vi "New Frame Trigger.vi"(8 "error in":errorcluster, 10 "Trigger":bool, 11 "CaptureDetectionLoopDataIn":T1={"Captures"=path "", "Timeout"=-1, "Reset"=TRUE, "Trigger"=FALSE, "Iteration"=0, "Capture"=path "", "Mode"=enum."Record", "Replay Run ID"=""}) -> (0 "error out":errorcluster, 2 "Latest Frame":path, 3 "CaptureDetectionLoopDataOut":T1={"Captures"=path "", "Timeout"=-1, "Reset"=TRUE, "Trigger"=FALSE, "Iteration"=0, "Capture"=path "", "Mode"=enum."Record", "Replay Run ID"=""})   [LabVIEW 2026, in "Launcher.lvlib"]
uses:
  Launcher.lvlib
  Capture detection loop data--cluster.ctl
  Mode.ctl
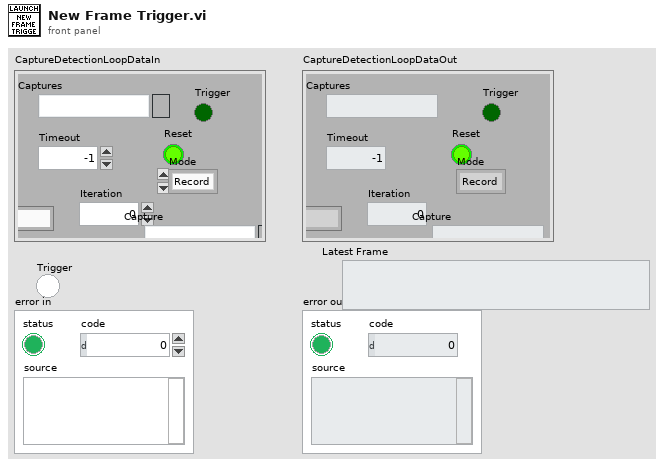
[diagram p1: front panel]
types:
  T1 = typedef "Capture detection loop data--cluster.ctl" = cluster{"Captures":path, "Timeout":i32, "Reset":bool, "Trigger":bool, "Iteration":i32, "Capture":path, "Mode":T2, "Replay Run ID":string}
  T2 = typedef "Mode.ctl" = enum16{"Record", "Record and Replay"}
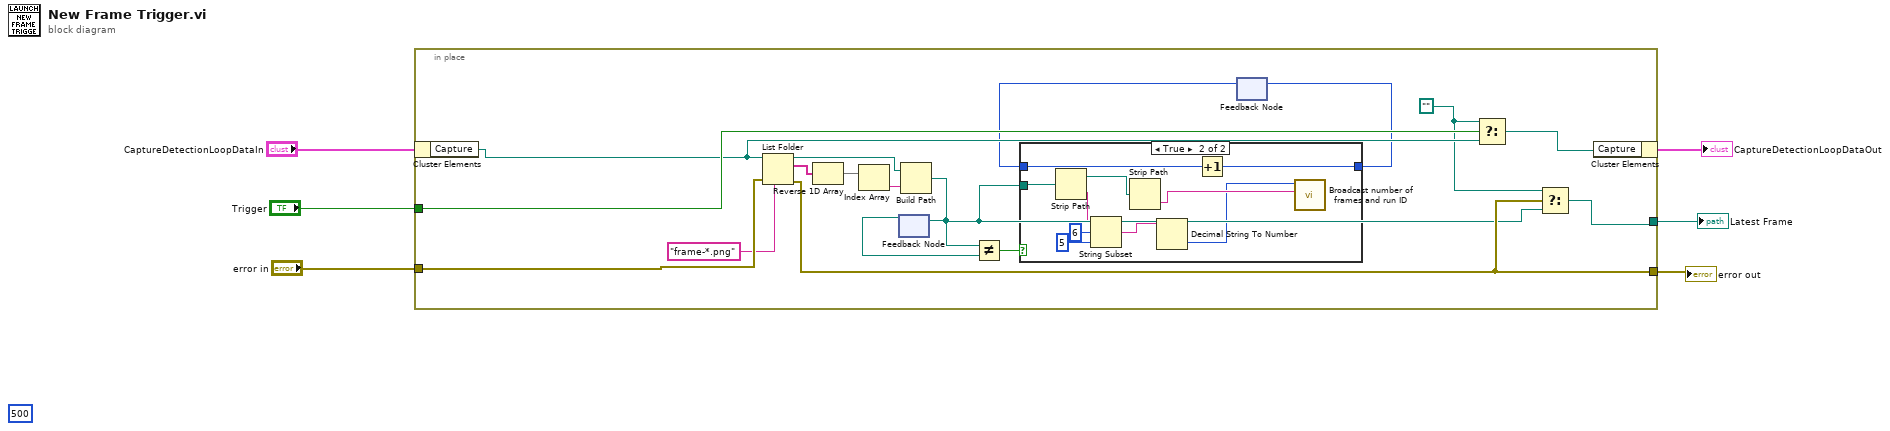
[diagram p0: block diagram]
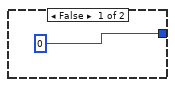
[diagram p2: hidden frame]
diagram:
  (unwired) 500
  n1 = in-place {
    in-place-border: [w15] -> w4
    in-place-border: "error in" -> [w22]
    in-place-border: [w14] -> w3
    in-place-border: "Trigger" -> [w17]
    w12 = path ""
    n2 = in-place-cluster #1("CaptureDetectionLoopDataIn") -> ("Capture"=w13:path)
    n3 = List Folder(path=w13, pattern="frame-*.png", error in=w22) -> (path out=w18:path, filenames=w16:string[], error out=w15:errorcluster)  [unwired: 1 in, 1 out]
    n4 = Reverse 1D Array(array=w16) -> (reversed array=w21:string[])
    n5 = Index Array(array=w21) -> (element=w20:string)  [unwired: 1 in]
    n6 = feedback #2() -> (w11:path)  [unwired: 1 in]
    n7 = Build Path(base path=w18, name or relative path=w20) -> (appended path=w9:path)
    n8 = feedback-in #2(w9) -> ()
    n9 = Not Equal?(x=w9, y=w11) -> (x != y?=w10:bool)
    n10 = feedback #3() -> (w7:u32)  [unwired: 1 in]
    n11 = case shown="True" w10 {
      tunnel: w9 -> [_ w34]
      tunnel: [u32 0 ("Number of frames") w30] -> w8
      tunnel: w7 -> [_ w31]
      frame False {
      }
      frame True {
        n12 = Strip Path(path=w34) -> (stripped path=w33:path, name=w29:string)
        n13 = String Subset(string=w29, offset (0)=6, length (rest)=5 ("length (rest)")) -> (substring=w26:string)
        n14 = Strip Path(path=w33) -> (name=w32:string)  [unwired: 1 out]
        n15 = Decimal String To Number(string=w26) -> (number=w25:i32)  [unwired: 2 in, 1 out]
        n16 = Increment(x=w31) -> (x+1=w30:u32)
        n17 = call "Broadcast number of frames and run ID.vi"("Run ID"=w32, "Number of frames"=w25) -> ()  [unwired: 9 in, 1 out]
      }
    }
    n18 = feedback-in #3(w8) -> ()
    n19 = Select(t=w12, s=w17, f=w13) -> (s? t:f=w23:path)
    n20 = Select(t=w12, s=w15, f=w9) -> (s? t:f=w14:path)
    n21 = in-place-cluster #1("Capture"=w23) -> (→"CaptureDetectionLoopDataOut":T1)
  }
  "error out" <- w4
  "Latest Frame" <- w3
